vi "FTW-Subscriber-AddAddresses.vi"(0 "FTW-Subscription In":refnum<class "FTW-Subscriber.lvclass">, 5 "Addresses":string, 11 "error in (no error)":errorcluster) -> (4 "FTW-Subscription Out":refnum<class "FTW-Subscriber.lvclass">, 15 "error out":errorcluster)   [LabVIEW 2013, in "FTW-Subscriber.lvclass"]
uses:
  FTW-Subscriber.lvclass
  FTW-Subscriber.lvclass/FTW-Subscriber.ctl
  Ether/FTW-Ether-EndpointType.ctl
  Endpoint/FTW-Endpoint.lvclass
  Ether/FTW-Ether.lvclass
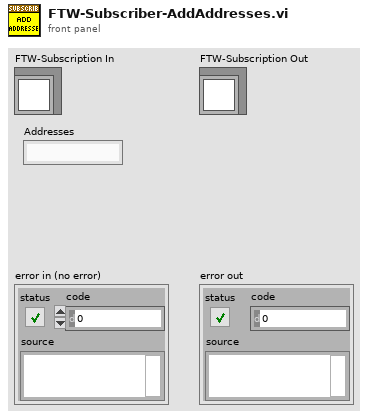
[diagram p1: front panel]
types:
  T1 = typedef "FTW-Ether.lvclass/FTW-Ether-EndpointType.ctl" = enum16{"Server", "Client", "Publisher", "Subscriber"}
  T2 = typedef "FTW-Ether.lvclass/FTW-Ether-MessageTransportScheme.ctl" = enum16{"LabVIEW Queues (lvq://)", "TCP (tcp://)"}
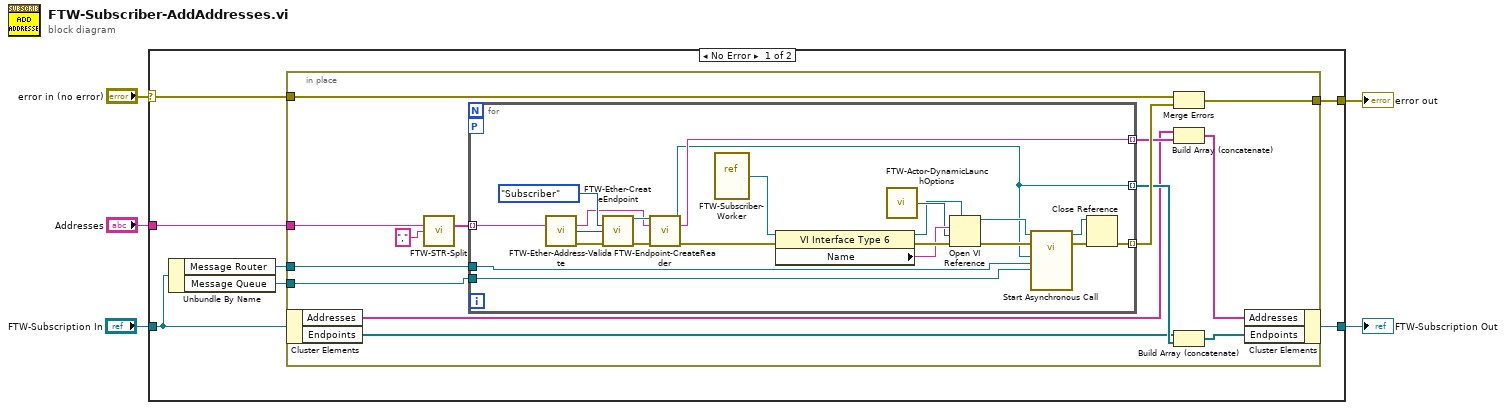
[diagram p0: block diagram]
diagram:
  n1 = case shown="No Error" "error in (no error)" {
    selector: "error in (no error)" -> [w12 w49]
    tunnel: [w11 w49] -> w4
    tunnel: "Addresses" -> [w10 _]
    tunnel: "FTW-Subscription In" -> [w8 w50]
    tunnel: [w9 w50] -> w1
    frame No Error {
      n2 = Unbundle By Name(w8) -> ("Message Router"=w7:refnum<user-event>, "Message Queue"=w6:refnum<queue>)
      n3 = in-place {
        in-place-border: w12 -> [w26]
        in-place-border: [w25] -> w11
        in-place-border: w10 -> [w22]
        in-place-border: w7 -> [w14]
        in-place-border: w6 -> [w13]
        n4 = in-place-cluster #1(w8) -> ("Addresses"=w16:string[], "Endpoints"=w15:refnum<class "FTW-Endpoint.lvclass">[])
        n5 = call "FTW-STR-Split.vi"("Delimited String"=w22, "Delimiter"=",") -> ("Array of Strings"=w24:string[])  [unwired: 13 in]
        n6 = for {
          tunnel: [w36] -> w21 mode=indexing
          tunnel: w24 -> [w35] mode=indexing
          tunnel: [w27] -> w19 mode=indexing
          tunnel: [w28] -> w20 mode=indexing
          workers-P: _ -> [_]
          tunnel: w14 -> [w34]
          tunnel: w13 -> [w33]
          n7 = call "FTW-Ether-Address-Validate.vi"("Address"=w35) -> ("Sanitized Address"=w29:string, "Message Transport Scheme"=w40:T2, "error out"=w38:errorcluster)  [unwired: 12 in]
          n8 = call "FTW-Ether-CreateEndpoint.vi"("Endpoint Type"=FTW-Ether-EndpointType."Subscriber", "Message Transport Scheme"=w40, "error in"=w38) -> ("FTW Endpoint"=w30:refnum<class "FTW-Endpoint.lvclass">, "error out"=w32:errorcluster)  [unwired: 11 in]
          n9 = call-dynamic "FTW-Endpoint-CreateReader.vi"("FTW-Endpoint In"=w30, "Address"=w29, "error in"=w32) -> ("FTW-Endpoint Out"=w27:refnum<class "FTW-Endpoint.lvclass">, "Actual Address"=w28:string, "error out"=w31:errorcluster)  [unwired: 10 in]
          n10 = vi-ref "FTW-Subscriber-Worker.vi"() -> (w48:refnum<vi>)
          n11 = property class="VI Interface Type 6"(reference=w48, error in=w31) -> (reference out=w44:refnum<vi>, error out=w47:errorcluster, "Name"=w46:string)
          n12 = call "FTW-Actor-DynamicLaunchOptions.vi"() -> ("Open VI Ref Options"=w45:i32)
          n13 = Open VI Reference(type specifier VI Refnum (for type only)=w44, vi path=w46, options=w45, error in (no error)=w47) -> (vi reference=w42:refnum<vi>, error out=w37:errorcluster)  [unwired: 2 in]
          n14 = call-by-ref "Start Asynchronous Call"(reference=w42, error in=w37, "Endpoint"=w27, "Message Handler"=w34, "Queue"=w33) -> (reference out=w41:refnum<vi>, error out=w43:errorcluster)  [unwired: 13 in]
          n15 = Close Reference(reference=w41, error in (no error)=w43) -> (error out=w36:errorcluster)
        }
        n16 = Merge Errors(w26, w21) -> (w25:errorcluster)
        n17 = Build Array (concatenate)(w16, w20) -> (w18:string[])
        n18 = Build Array (concatenate)(w15, w19) -> (w17:refnum<class "FTW-Endpoint.lvclass">[])
        n19 = in-place-cluster #1("Addresses"=w18, "Endpoints"=w17) -> (w9:refnum<class "FTW-Subscriber.lvclass">)
      }
    }
    frame Error {
    }
  }
  "error out" <- w4
  "FTW-Subscription Out" <- w1
